vi "PH_Tektronix_7000.Configure Acquisition.vi"(0 "i ref in":refnum<vi>, 2 "Acquisition Configuration":T1={"Record Length"=10000, "Timebase [s/div]"=4.0, "Position [%]"=0.0, "Acquisition Type"=0, "Average Waveforms"=10, "Envelope Waveforms"=10, "WfmDB Samples"=16000, "Continuous?"=FALSE, "Delay [s]"=0.0, "Run?"=FALSE} {"Delay [s]" format="%#_12p"; "Acquisition Type" items=["Sample", "Peak Detect", "Hi Res", "Average", "Envelope", "WfmDB"]; "Timebase [s/div]" format="%#_12g"}, 5 "error IO":errorcluster) -> (14 "i ref out":refnum<vi>, 19 "error out":errorcluster)   [LabVIEW 2014, in "PH_Tektronix_7000.lvlib"]
doc: "If the connection is established, the acquisition configuration is set and written to own attributes as well as the errors."
uses:
  PH_Tektronix_7000.lvlib
  PH_Tektronix_7000.Acquisition Config.ctl
  instr.lib/Tektronix7000Series/Tektronix 7000 Series - Driver np.lvlib
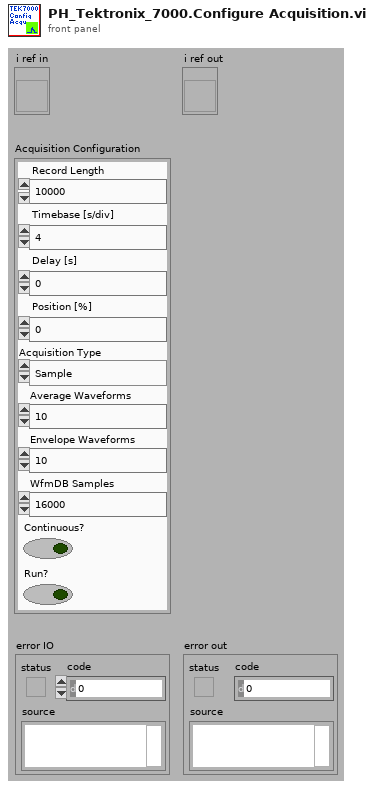
[diagram p1: front panel]
types:
  T1 = typedef "PH_Tektronix_7000.lvlib/PH_Tektronix_7000.Acquisition Config.ctl" = cluster{"Record Length":u32, "Timebase [s/div]":dbl, "Position [%]":dbl, "Acquisition Type":u16, "Average Waveforms":i32, "Envelope Waveforms":i32, "WfmDB Samples":i32, "Continuous?":bool, "Delay [s]":dbl, "Run?":bool}
  T2 = typedef "PH_Tektronix_7000.lvlib/PH_Tektronix_7000.i attribute.ctl" = cluster{"VISA Resource Name":refnum<visa-resource-name>, "IDN":cluster{"Instrument Driver":string, "Instrument Firmware":string, "Model":string, "Serial Number":string}, "Selftest":cluster{"Result":i32, "Message":string}, "Trigger Configuration":T3, "Acquisition Configuration":T1, "GUI Refs":T4, "State":T5, "Error Message":string, "Allow Prdc Loop?":bool, "Channel 1":T6, "Channel 2":T6, "Channel 3":T6, "Channel 4":T6, "Data CH 1":waveform(dbl), "Data CH 2":waveform(dbl), "Data CH 3":waveform(dbl), "Data CH 4":waveform(dbl), "Allow config?":bool, "Name Channel 1":string, "Name Channel 2":string, "Name Channel 3":string, "Name Channel 4":string, "Fetch Data before sending to PSDB?":bool, "Constructor passed?":bool, "Data taken at":timestamp, "Plot Colors":u32[], "Default VISA Resource":string}
  T3 = typedef "PH_Tektronix_7000.lvlib/PH_Tektronix_7000.Trigger Config.ctl" = cluster{"Source":u16, "Level [V]":dbl, "Slope":u16, "Coupling":u16, "Trigger Mode":u16}
  T4 = typedef "PH_Tektronix_7000.lvlib/PH_Tektronix_7000.GUI Refs.ctl" = cluster{"Graph":refnum<vi>, "State":refnum<vi>, "Delete":refnum<vi>, "VISA Resource":refnum<vi>, "Allow Configure":refnum<vi>, "Fetch Data":refnum<vi>, "Fetch before sending Data to PSDB":refnum<vi>, "Name Channel 1":refnum<vi>, "Name Channel 2":refnum<vi>, "Name Channel 3":refnum<vi>, "Name Channel 4":refnum<vi>, "Prdc Intervall [ms]":refnum<vi>, "Data taken":refnum<vi>, "Model":refnum<vi>, "Serial Number":refnum<vi>, "Firmware":refnum<vi>, "Driver":refnum<vi>, "Acquisition":refnum<vi>, "Trigger":refnum<vi>, "Cursor: D Time [s]":refnum<vi>, "Cursor: D Signal [V]":refnum<vi>, "Channel 1":refnum<vi>, "Channel 2":refnum<vi>, "Channel 3":refnum<vi>, "Channel 4":refnum<vi>}
  T5 = typedef "PH_StatusHandler.lvlib/PH_StatusHandler.Status.ctl" = i16
  T6 = typedef "PH_Tektronix_7000.lvlib/PH_Tektronix_7000.Channel Config.ctl" = cluster{"Enable Channel":bool, "Bandwidth":u16, "Input Impedance":u16, "Vertical Coupling":u16, "Probe Attenuation":dbl, "Range [V/div]":dbl, "Position [div]":dbl, "Bandwidth raw":string}
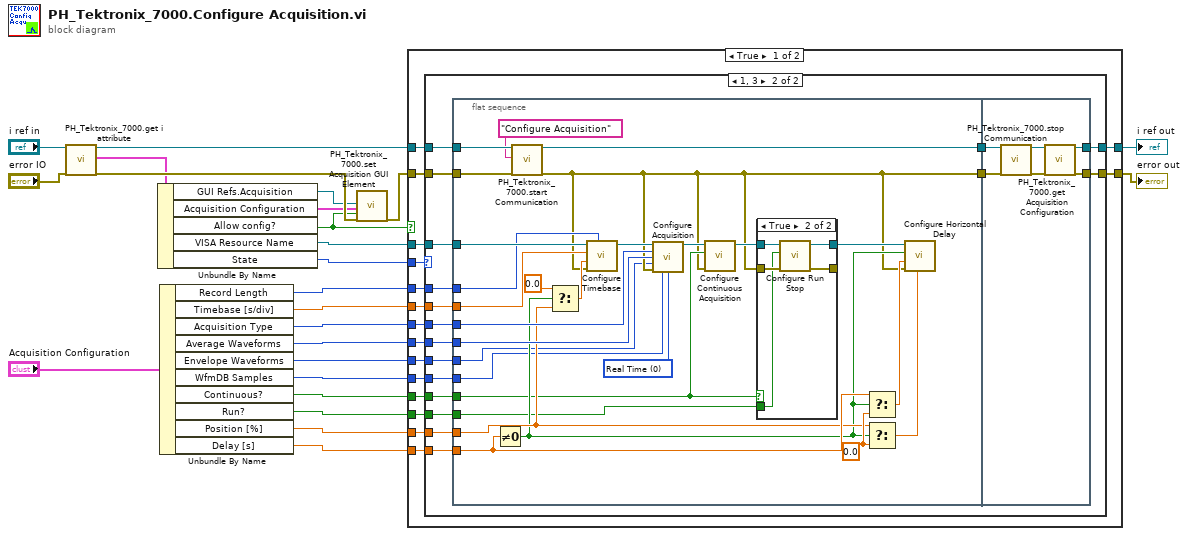
[diagram p0: block diagram]
diagram:
  n1 = call "PH_Tektronix_7000.get i attribute.vi"("i ref in"="i ref in", "error in (no error)"="error IO") -> ("i ref out"=w16:refnum<vi>, "i attribute"=w17:T2, "error out"=w19:errorcluster)  [unwired: 15 in]
  n2 = Unbundle By Name(w17) -> ("GUI Refs.Acquisition"=w2:refnum<vi>, "Acquisition Configuration"=w4:T1, "Allow config?"=w3:bool, "VISA Resource Name"=w18:refnum<visa-resource-name>, "State"=w11:T5)
  n3 = Unbundle By Name("Acquisition Configuration") -> ("Record Length"=w15:u32, "Timebase [s/div]"=w14:dbl, "Acquisition Type"=w13:u16, "Average Waveforms"=w12:i32, "Envelope Waveforms"=w10:i32, "WfmDB Samples"=w9:i32, "Continuous?"=w8:bool, "Run?"=w1:bool, "Position [%]"=w6:dbl, "Delay [s]"=w7:dbl)
  n4 = call "PH_Tektronix_7000.set Acquisition GUI Element.vi"("Ref Acqu Config"=w2, "Acqu Config"=w4, "enabled?"=w3, "error in"=w19) -> ("error out"=w5:errorcluster)  [unwired: 15 in]
  n5 = case shown="True" w3 {
    tunnel: [w40 w101] -> w24
    tunnel: [w39 w100] -> w23
    tunnel: w5 -> [w38 w100]
    tunnel: w18 -> [w37 _]
    tunnel: w16 -> [w36 w101]
    tunnel: w15 -> [w35 _]
    tunnel: w14 -> [w34 _]
    tunnel: w6 -> [w33 _]
    tunnel: w13 -> [w32 _]
    tunnel: w12 -> [w31 _]
    tunnel: w11 -> [w30 _]
    tunnel: w10 -> [w29 _]
    tunnel: w9 -> [w28 _]
    tunnel: w8 -> [w27 _]
    tunnel: w7 -> [w26 _]
    tunnel: w1 -> [w25 _]
    frame True {
      n6 = case shown="1, 3" w30 {
        tunnel: w36 -> [w42 w58]
        tunnel: w37 -> [_ w57]
        tunnel: [w41 w45] -> w39
        tunnel: w38 -> [w41 w59]
        tunnel: [w42 w46] -> w40
        tunnel: w35 -> [_ w56]
        tunnel: w34 -> [_ w55]
        tunnel: w33 -> [_ w49]
        tunnel: w32 -> [_ w54]
        tunnel: w31 -> [_ w53]
        tunnel: w29 -> [_ w52]
        tunnel: w28 -> [_ w51]
        tunnel: w27 -> [_ w47]
        tunnel: w26 -> [_ w50]
        tunnel: w25 -> [_ w48]
        frame Default {
        }
        frame 1, 3 {
          n7 = flat-sequence {
            tunnel: w59 -> [w86]
            tunnel: w58 -> [w85]
            tunnel: w57 -> [w83]
            tunnel: w56 -> [w82]
            tunnel: w55 -> [w81]
            tunnel: w54 -> [w79]
            tunnel: w53 -> [w78]
            tunnel: w52 -> [w60]
            tunnel: w51 -> [w61]
            tunnel: w50 -> [w73]
            tunnel: w49 -> [w70]
            tunnel: w48 -> [w66]
            tunnel: w47 -> [w65]
            tunnel: [w64] -> w44
            tunnel: [w63] -> w43
            tunnel: [w97] -> w45
            tunnel: [w99] -> w46
            tunnel: w44 -> [w95]
            tunnel: w43 -> [w98]
            frame #0 {
              w62 = u16 0 items=["Real Time", "Interpolater", "Equivalent"] ("Sampling Modes (Real Time)")
              w71 = 0.0 ("f")
              n8 = Not Equal To 0?(x=w73) -> (x != 0?=w69:bool)
              n9 = call "PH_Tektronix_7000.start Communication.vi"("i ref in"=w85, "Action"="Configure Acquisition", "error in"=w86) -> ("i ref out"=w64:refnum<vi>, "error out"=w63:errorcluster)  [unwired: 15 in]
              n10 = Select(t=0.0 ("f"), s=w69, f=w70) -> (s? t:f=w74:dbl)
              n11 = call "Configure Timebase.vi"("Record Length (10000)"=w82, "error in (no error)"=w63, "Position (0.0 s)"=w74, "Timebase (1e-9s)"=w81, "VISA resource name"=w83) -> ("VISA resource name out"=w80:refnum<visa-resource-name>)  [unwired: 5 in, 1 out]
              n12 = call "Configure Acquisition.vi"("VISA resource name"=w80, "Acquisition Type (0:Sample)"=w79, "Average Waveforms (10)"=w78, "Envelope Waveforms (10)"=w60, "error in (no error)"=w63, "WfmDB Samples (16000)"=w61, "Sampling Modes (Real Time)"=w62) -> ("VISA resource name out"=w77:refnum<visa-resource-name>)  [unwired: 7 in, 1 out]
              n13 = call "Configure Continuous Acquisition.vi"("error in (no error)"=w63, "Enable Continuous Acquisition Mode (True)"=w65, "VISA resource name"=w77) -> ("VISA resource name out"=w68:refnum<visa-resource-name>)  [unwired: 7 in, 1 out]
              n14 = case shown="True" w65 {
                tunnel: w63 -> [w87 w93]
                tunnel: [w87 w92] -> _
                tunnel: w68 -> [w88 w91]
                tunnel: [w88 w90] -> w67
                tunnel: w66 -> [_ w89]
                frame False {
                }
                frame True {
                  n15 = call "Configure Run Stop.vi"("error in (no error)"=w93, "Enable Continuous Acquisition Mode (True)"=w89, "VISA resource name"=w91) -> ("error out"=w92:errorcluster, "VISA resource name out"=w90:refnum<visa-resource-name>)  [unwired: 7 in]
                }
              }
              n16 = Select(t=w73, s=w69, f=w71) -> (s? t:f=w72:dbl)
              n17 = Select(t=w70, s=w69, f=w71) -> (s? t:f=w76:dbl)
              n18 = call "Configure Horizontal Delay.vi"("Position [s]"=w76, "error in (no error)"=w63, "Delay [s]"=w72, "Activate Delay?"=w69, "VISA resource name"=w67) -> ()  [unwired: 5 in, 2 out]
            }
            frame #1 {
              n19 = call "PH_Tektronix_7000.stop Communication.vi"("i ref in"=w95, "error in"=w98) -> ("i ref out"=w94:refnum<vi>, "error out"=w96:errorcluster)  [unwired: 16 in]
              n20 = call "PH_Tektronix_7000.get Acquisition Configuration.vi"("i ref in"=w94, "error IO"=w96) -> ("i ref out"=w99:refnum<vi>, "error out"=w97:errorcluster)  [unwired: 16 in]
            }
          }
        }
      }
    }
    frame False {
    }
  }
  "i ref out" <- w24
  "error out" <- w23
